vi "fix_null_ranges.vi"(11 "input cluster":T1) -> (3 "output cluster":T1)   [LabVIEW 2020, in "3DPC_SurfacePlot.xctl"]
uses:
  <vilib>/Native 3D Graph/xcontrol/3DPC_SurfacePlot.xctl
  <vilib>/Native 3D Graph/typedefs/range_cluster.ctl
  <vilib>/Native 3D Graph/typedefs/min_max.ctl
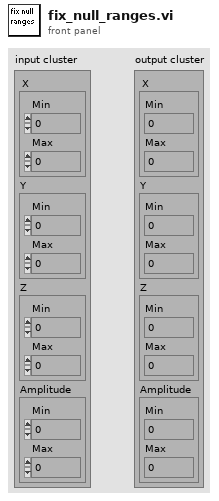
[diagram p1: front panel]
types:
  T1 = typedef "3DPC_SurfacePlot.xctl/range_cluster.ctl" = cluster{"X":T2, "Y":T2, "Z":T2, "Amplitude":T2}
  T2 = typedef "3DPC_SurfacePlot.xctl/min_max.ctl" = cluster{"Min":sgl, "Max":sgl}
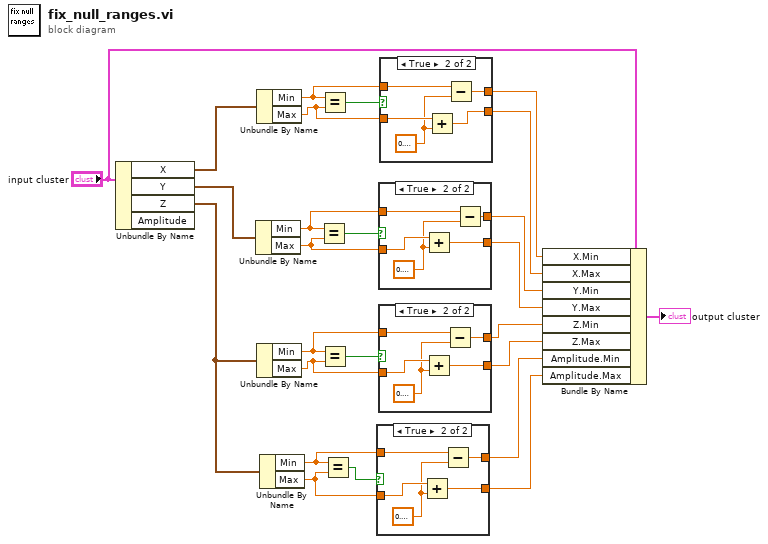
[diagram p0: block diagram]
diagram:
  n1 = Unbundle By Name("input cluster") -> ("X"=w25:T2, "Y"=w20:T2, "Z"=w14:T2)  [unwired: 1 out]
  n2 = Unbundle By Name(w20) -> ("Min"=w6:sgl, "Max"=w18:sgl)
  n3 = Unbundle By Name(w25) -> ("Min"=w8:sgl, "Max"=w23:sgl)
  n4 = Unbundle By Name(w14) -> ("Min"=w3:sgl, "Max"=w17:sgl)
  n5 = Unbundle By Name(w14) -> ("Min"=w1:sgl, "Max"=w13:sgl)
  n6 = Equal?(x=w6, y=w18) -> (x = y?=w19:bool)
  n7 = Equal?(x=w8, y=w23) -> (x = y?=w24:bool)
  n8 = Equal?(x=w3, y=w17) -> (x = y?=w16:bool)
  n9 = Equal?(x=w1, y=w13) -> (x = y?=w15:bool)
  n10 = case shown="True" w15 {
    tunnel: w13 -> [w27 w32]
    tunnel: [w27 w31] -> w9
    tunnel: [w26 w30] -> w2
    tunnel: w1 -> [w26 w29]
    frame False {
    }
    frame True {
      w28 = sgl 0.1 ("y")
      n11 = Add(x=w32, y=w28) -> (x+y=w31:sgl)
      n12 = Subtract(x=w29, y=w28) -> (x-y=w30:sgl)
    }
  }
  n13 = case shown="True" w19 {
    tunnel: w18 -> [w34 w39]
    tunnel: [w34 w38] -> w11
    tunnel: w6 -> [w33 w37]
    tunnel: [w33 w36] -> w5
    frame False {
    }
    frame True {
      w35 = sgl 0.1 ("y")
      n14 = Add(x=w39, y=w35) -> (x+y=w38:sgl)
      n15 = Subtract(x=w37, y=w35) -> (x-y=w36:sgl)
    }
  }
  n16 = case shown="True" w16 {
    tunnel: w17 -> [w41 w46]
    tunnel: [w41 w45] -> w10
    tunnel: [w40 w44] -> w4
    tunnel: w3 -> [w40 w43]
    frame False {
    }
    frame True {
      w42 = sgl 0.1 ("y")
      n17 = Add(x=w46, y=w42) -> (x+y=w45:sgl)
      n18 = Subtract(x=w43, y=w42) -> (x-y=w44:sgl)
    }
  }
  n19 = case shown="True" w24 {
    tunnel: w23 -> [w48 w53]
    tunnel: [w48 w52] -> w21
    tunnel: w8 -> [w47 w51]
    tunnel: [w47 w50] -> w7
    frame False {
    }
    frame True {
      w49 = sgl 0.1 ("y")
      n20 = Add(x=w53, y=w49) -> (x+y=w52:sgl)
      n21 = Subtract(x=w51, y=w49) -> (x-y=w50:sgl)
    }
  }
  n22 = Bundle By Name(cluster="input cluster", "X.Min"=w7, "X.Max"=w21, "Y.Min"=w5, "Y.Max"=w11, "Z.Min"=w4, "Z.Max"=w10, "Amplitude.Min"=w2, "Amplitude.Max"=w9) -> (→"output cluster":T1)
